vi "VI Server_Get TabControl Cluster.vi"(7 "TabControl Label":string, 8 "error in":errorcluster, 11 "VI Server Cluster":T1) -> (0 "error out":errorcluster, 3 "VI Server Cluster.OUT":T1)   [LabVIEW 2020, in "VI Server Toolkit LV2013.lvlib"]
doc: "Extracts control labels and references containing in a tab control and merges onto incoming VI server Cluster."
uses:
  VI Server Toolkit LV2013.lvlib
  VI Server_TypeDefs/VI Server_RefsCluster.ctl
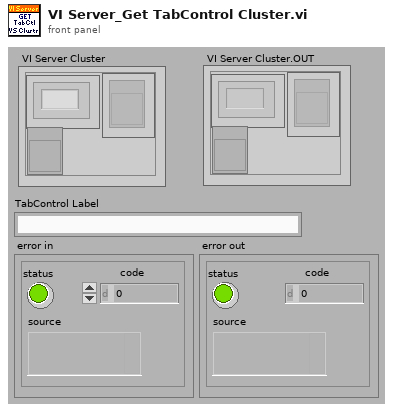
[diagram p1: front panel]
types:
  T1 = typedef "VI Server_RefsCluster.ctl" = cluster{"Labels":string[], "Refs":refnum<vi>[], "VI Ref":refnum<vi>}
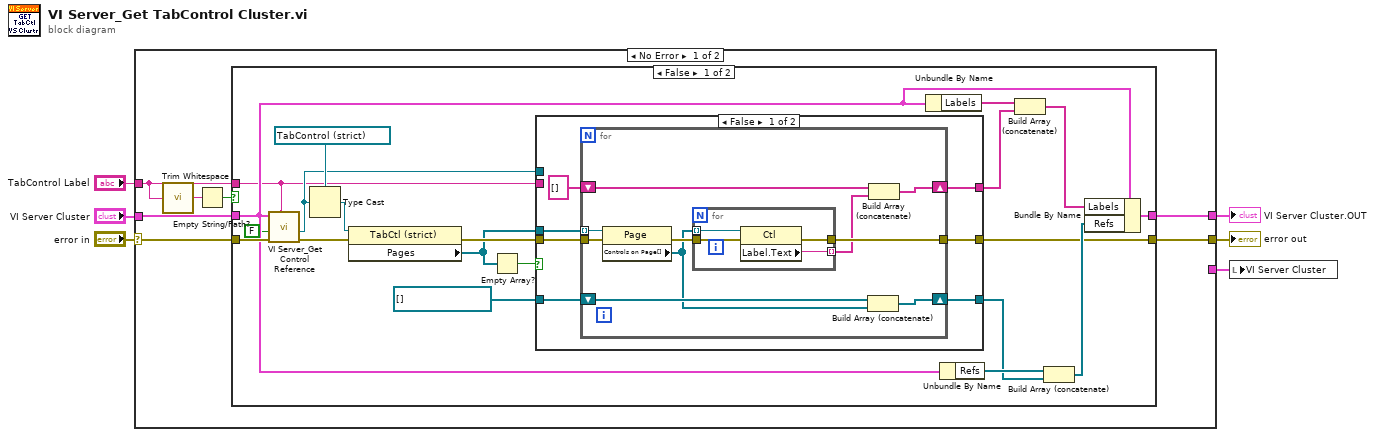
[diagram p0: block diagram]
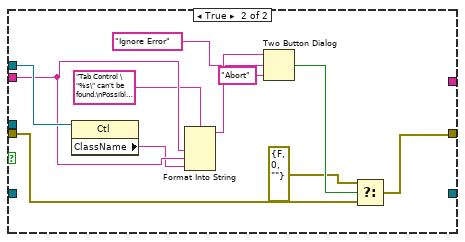
[diagram p2: hidden frame]
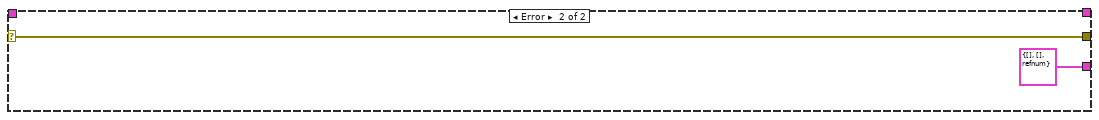
[diagram p4: hidden frame]
diagram:
  n1 = case shown="No Error" "error in" {
    selector: "error in" -> [w12 w69]
    tunnel: "VI Server Cluster" -> [w11 _]
    tunnel: [w13 w69] -> w5
    tunnel: [w8 _] -> w3
    tunnel: "TabControl Label" -> [w7 _]
    tunnel: [_ T1 {"Labels"=[], "Refs"=[], "VI Ref"=refnum} ("VI Server Cluster")] -> w1
    frame No Error {
      n2 = call <vilib>:"Trim Whitespace.vi"("string"=w7) -> ("trimmed string"=w10:string)  [unwired: 1 in]
      n3 = Empty String/Path?(string/path=w10) -> (empty?=w9:bool)
      n4 = case shown="False" w9 {
        tunnel: [w18 w67] -> w13
        tunnel: w12 -> [w33 w67]
        tunnel: w11 -> [w27 w66]
        tunnel: [w24 w66] -> w8
        tunnel: w7 -> [w14 _]
        frame False {
          n5 = call "VI Server_Get Control Reference.vi"("Label"=w14, "error in"=w33, "Single Instance (T)"=FALSE, "VI Server Cluster"=w27) -> ("error out"=w32:errorcluster, "Control Reference (Generic)"=w16:refnum<vi>)  [unwired: 6 out]
          n6 = Type Cast(type=refnum<vi> refnum ("TabCtlRef"), x=w16) -> (*(type *) &x=w17:refnum<vi>)
          n7 = property class="TabCtl (strict)"(reference=w17, error in=w32) -> (error out=w31:errorcluster, "Pages"=w21:refnum<vi>[])  [unwired: 1 out]
          n8 = Empty Array?(array=w21) -> (empty?=w20:bool)
          n9 = case shown="False" w20 {
            tunnel: [w40 w56] -> w18
            tunnel: w31 -> [w39 w57]
            tunnel: refnum<vi>[] [] ("Controls on Page[]") -> [w37 _]
            tunnel: [w36 _] -> w23
            tunnel: [w35 _] -> w19
            tunnel: w21 -> [w34 _]
            tunnel: w14 -> [_ w63]
            tunnel: w16 -> [_ w64]
            frame False {
              n10 = for {
                tunnel: w39 -> [w49]
                tunnel: [w47] -> w40
                tunnel: w34 -> [w50] mode=indexing
                shift-right: [w41] -> w35
                shift-left: string[] [] -> [w46]
                shift-right: [w43] -> w36
                shift-left: w37 -> [w44]
                n11 = property class="Page"(reference=w50, error in=w49) -> (error out=w48:errorcluster, "Controls on Page[]"=w42:refnum<vi>[])  [unwired: 1 out]
                n12 = for {
                  tunnel: w48 -> [w54]
                  tunnel: w42 -> [w53] mode=indexing
                  tunnel: [w52] -> w47
                  tunnel: [w51] -> w45 mode=indexing
                  n13 = property class="Ctl"(reference=w53, error in=w54) -> (error out=w52:errorcluster, "Label.Text"=w51:string)  [unwired: 1 out]
                }
                n14 = Build Array (concatenate)(w44, w42) -> (w43:refnum<vi>[])
                n15 = Build Array (concatenate)(w46, w45) -> (w41:string[])
              }
            }
            frame True {
              n16 = property class="Ctl"(reference=w64) -> ("ClassName"=w62:string)  [unwired: 1 in, 2 out]
              n17 = Format Into String(format string="Tab Control \"%s\" can't be found.\nPossible reason:\n1. Wrong name.\n2. It is part of another\nstacked structure.\n3. Control Label \"%s\" being entered for the tab is actually referencing to %s Class ID.", w63, w63, w62) -> (resulting string=w65:string)  [unwired: 2 in, 1 out]
              n18 = Two Button Dialog(message=w65, 1:"Abort" ("F button name (\"Cancel\")"), 2:"Ignore Error" ("T button name (\"OK\")")) -> (T button?=w58:bool)
              n19 = Select(t=errorcluster {"status"=FALSE, "code"=0, "source"=""}, s=w58, f=w57) -> (s? t:f=w56:errorcluster)
            }
          }
          n20 = Unbundle By Name(w27) -> ("Labels"=w29:string[])
          n21 = Unbundle By Name(w27) -> ("Refs"=w28:refnum<vi>[])
          n22 = Build Array (concatenate)(w29, w19) -> (w26:string[])
          n23 = Build Array (concatenate)(w28, w23) -> (w25:refnum<vi>[])
          n24 = Bundle By Name(cluster=w27, "Labels"=w26, "Refs"=w25) -> (w24:T1)
        }
        frame True {
        }
      }
    }
    frame Error {
    }
  }
  "error out" <- w5
  "VI Server Cluster.OUT" <- w3
  n25 = local write "VI Server Cluster"(w1) -> ()
